vi "CycleHistoryBufferStatus.vi"(8 "error in (no error)":errorcluster, 11 "ERD Data In":T2[](array[typedef]) {"ERD Number" format="%.0x"}) -> (0 "error out":errorcluster, 3 "Cycle History Buffer Status":T1)   [LabVIEW 2016]
uses:
  Common/LabVIEW GEA2 Toolkit/LabVIEW_GEA2_Toolkit.lvlibp/type defs/ERD Read Data Out.ctl
  type defs/CycleHistoryBufferStatusTypeDef.ctl
  Common/LabVIEW GEA2 Toolkit/LabVIEW_GEA2_Toolkit.lvlibp
panel:
  # "Note: Error terminals are wired together, so VI\nwon't create any new errors, just pass existing ones."
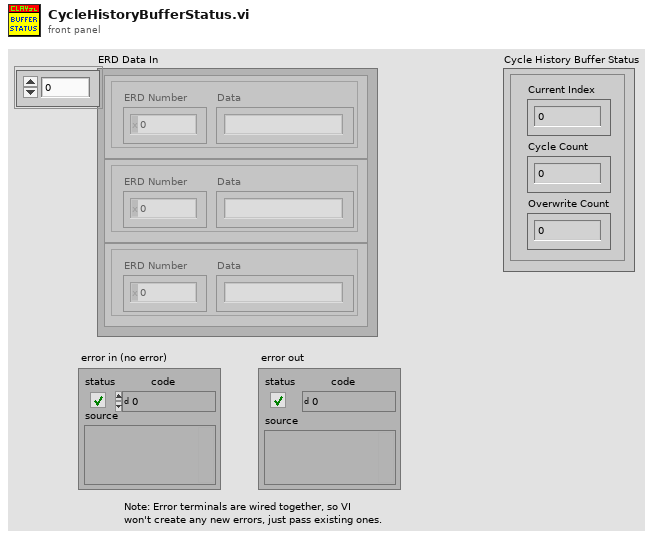
[diagram p1: front panel]
types:
  T1 = typedef "CycleHistoryBufferStatusTypeDef.ctl" = cluster{"Current Index":u16, "Cycle Count":u16, "Overwrite Count":u16}
  T2 = typedef "LabVIEW_GEA2_Toolkit.lvlibp/ERD Read Data Out.ctl" = cluster{"ERD Number":u16, "Data":string}
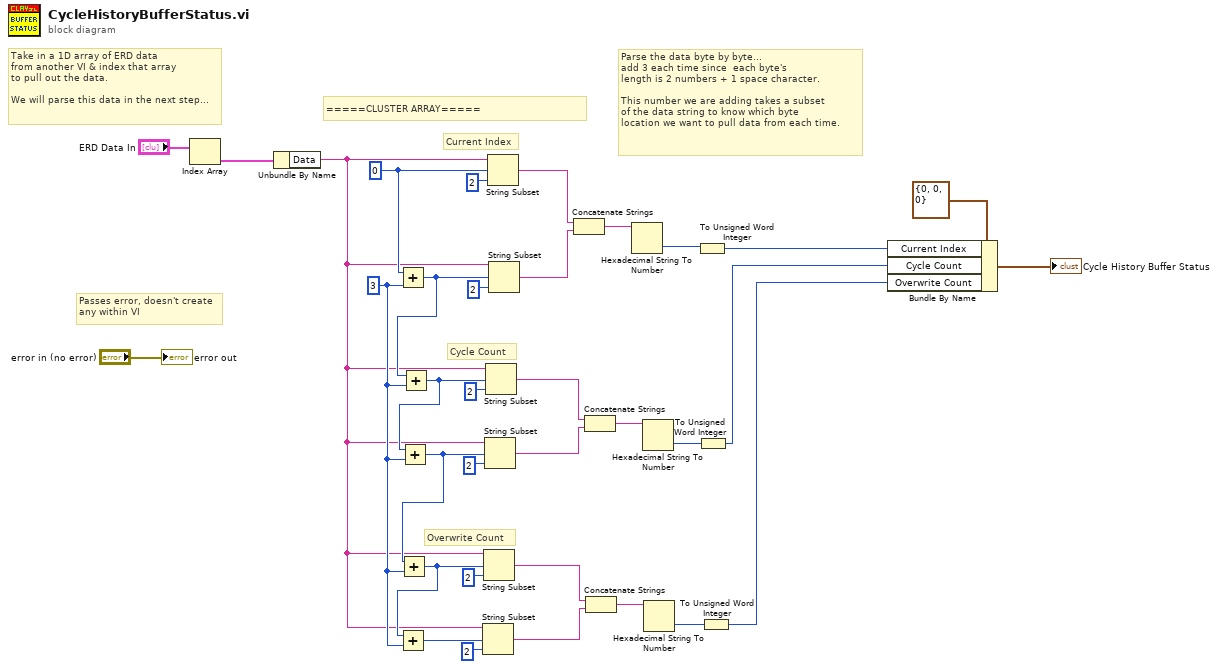
[diagram p0: block diagram]
diagram:
  w19 = 3 ("length (rest)")
  w30 = 0 ("offset (0)")
  # "=====CLUSTER ARRAY====="
  # "Parse the data byte by byte...\nadd 3 each time since  each byte's\nlength is 2 numbers + 1 space character.\n\nThis number we are adding takes a subset\nof the data string to know which byte\nlocation we want to pull data from each time."
  # "Take in a 1D array of ERD data\nfrom another VI & index that array\nto pull out the data. \n\nWe will parse this data in the next step..."
  # "Overwrite Count"
  # "Cycle Count"
  # "Current Index"
  # "Passes error, doesn't create\nany within VI"
  n1 = Index Array(array="ERD Data In") -> (element=w33:T2)  [unwired: 1 in]
  n2 = Unbundle By Name(w33) -> ("Data"=w18:string)
  n3 = Add(x=w30, y=w19) -> (x+y=w27:i32)
  n4 = Add(x=w27, y=w19) -> (x+y=w25:i32)
  n5 = Add(x=w25, y=w19) -> (x+y=w21:i32)
  n6 = Add(x=w21, y=w19) -> (x+y=w22:i32)
  n7 = Add(x=w22, y=w19) -> (x+y=w20:i32)
  n8 = String Subset(string=w18, offset (0)=w20, length (rest)=2 ("length (rest)")) -> (substring=w9:string)
  n9 = String Subset(string=w18, offset (0)=w22, length (rest)=2 ("length (rest)")) -> (substring=w10:string)
  n10 = String Subset(string=w18, offset (0)=w21, length (rest)=2 ("length (rest)")) -> (substring=w12:string)
  n11 = String Subset(string=w18, offset (0)=w25, length (rest)=2 ("length (rest)")) -> (substring=w13:string)
  n12 = String Subset(string=w18, offset (0)=w30, length (rest)=2 ("length (rest)")) -> (substring=w17:string)
  n13 = String Subset(string=w18, offset (0)=w27, length (rest)=2 ("length (rest)")) -> (substring=w16:string)
  n14 = Concatenate Strings(w17, w16) -> (w15:string)
  n15 = Concatenate Strings(w13, w12) -> (w14:string)
  n16 = Concatenate Strings(w10, w9) -> (w11:string)
  n17 = Hexadecimal String To Number(string=w15) -> (number=w8:u32)  [unwired: 2 in, 1 out]
  n18 = Hexadecimal String To Number(string=w14) -> (number=w7:u32)  [unwired: 2 in, 1 out]
  n19 = Hexadecimal String To Number(string=w11) -> (number=w6:u32)  [unwired: 2 in, 1 out]
  n20 = To Unsigned Word Integer(number=w8) -> (unsigned 16bit integer=w4:u16)
  n21 = To Unsigned Word Integer(number=w7) -> (unsigned 16bit integer=w3:u16)
  n22 = To Unsigned Word Integer(number=w6) -> (unsigned 16bit integer=w2:u16)
  n23 = Bundle By Name(cluster=T1 {"Current Index"=0, "Cycle Count"=0, "Overwrite Count"=0} ("Cycle History Buffer Status"), "Current Index"=w4, "Cycle Count"=w3, "Overwrite Count"=w2) -> (→"Cycle History Buffer Status":T1)
  "error out" <- "error in (no error)"
